vi "ExSubAsyncColDispStr.vi"(2 "error in (no error)":errorcluster, 3 "Store Data":bool, 4 "Display Title":string, 5 "Handle Cluster":T1) -> (0 "error out":errorcluster, 1 "Handle Cluster Out":T1)   [LabVIEW 2010]
panel:
  # "ExSubAsyncColDispStr:\nThis Sub-VI does the data collection, \ndisplay, and storage for Async\ncamera operations."
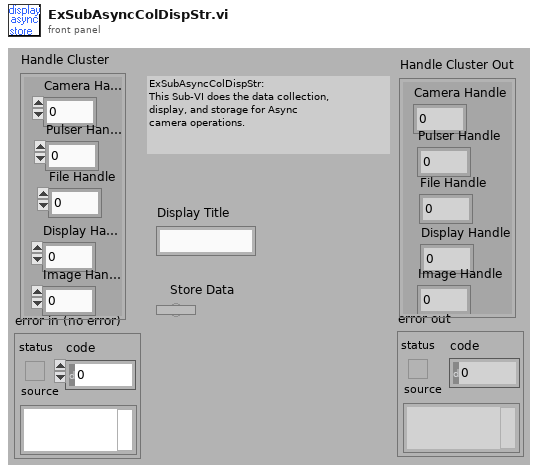
[diagram p1: front panel]
types:
  T1 = cluster{"Camera Handle":u32, "Pulser Handle":u32, "File Handle":u32, "Display Handle":u32, "Image Handle":u32}
  T2 = cluster{"Camera Handle":u32, "Pulser Handle":u32, "File Handle":u32, "Display Handle":u32, "Data Handle":u32}
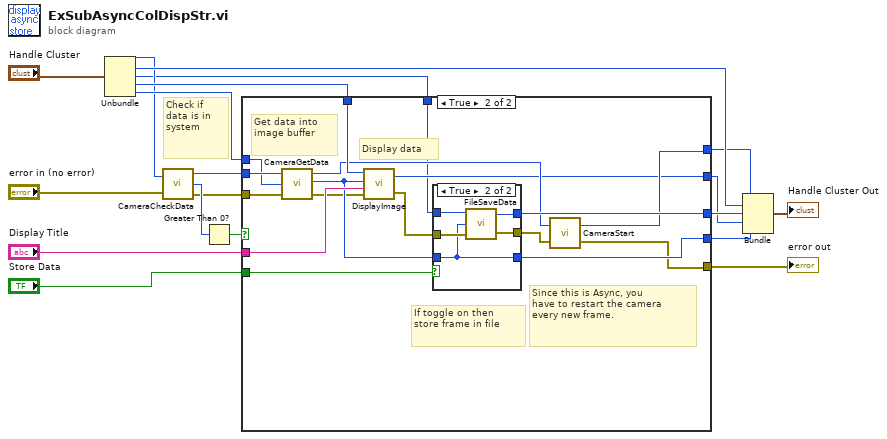
[diagram p0: block diagram]
diagram:
  # "Check if \ndata is in\nsystem"
  n1 = Unbundle("Handle Cluster") -> ("Camera Handle"=w6:u32, "Pulser Handle"=w9:u32, "File Handle"=w1:u32, "Display Handle"=w11:u32, "Image Handle"=w12:u32)
  n2 = call <userlib>:"CameraCheckData.vi"("Camera Handle"=w6, "error in"="error in (no error)") -> ("Camera Handle"=w16:u32, "Number Of Frames Available"=w15:i32, "error out"=w14:errorcluster)
  n3 = Greater Than 0?(x=w15) -> (x > 0?=w17:bool)
  n4 = case shown="True" w17 {
    tunnel: w16 -> [w24 w41]
    tunnel: w14 -> [w23 w40]
    tunnel: w12 -> [w21 w38]
    tunnel: w11 -> [w22 w37]
    tunnel: [w24 w28] -> w7
    tunnel: [w20 w39] -> w5
    tunnel: "Display Title" -> [_ w36]
    tunnel: w1 -> [w20 w25]
    tunnel: [w22 w26] -> w4
    tunnel: [w23 w29] -> w8
    tunnel: [w21 w34] -> w3
    tunnel: "Store Data" -> [_ w33]
    frame False {
    }
    frame True {
      # "If toggle on then\nstore frame in file"
      # "Since this is Async, you\nhave to restart the camera\nevery new frame."
      # "Display data"
      # "Get data into\nimage buffer"
      n5 = call <userlib>:"CameraGetData.vi"("error in"=w40, "Data Handle"=w38, "Camera Handle"=w41) -> ("error out"=w32:errorcluster, "Data Handle"=w35:u32, "Camera Handle"=w27:u32)
      n6 = call <userlib>:"DisplayImage.vi"("error in"=w32, "Title"=w36, "Image Handle"=w35, "Display Handle"=w37) -> ("error out"=w31:errorcluster, "Display Handle"=w26:u32)
      n7 = case shown="True" w33 {
        tunnel: [w44 w49] -> w39
        tunnel: w31 -> [w43 w48]
        tunnel: w25 -> [w44 w45]
        tunnel: [w43 w47] -> w30
        tunnel: w35 -> [w42 w46]
        tunnel: [w42 w46] -> w34
        frame False {
        }
        frame True {
          n8 = call <userlib>:"FileSaveData.vi"("error in"=w48, "Image Handle"=w46, "File Handle"=w45) -> ("error out"=w47:errorcluster, "File Handle"=w49:u32)
        }
      }
      n9 = call <userlib>:"CameraStart.vi"("error in"=w30, "Camera Handle"=w27) -> ("error out"=w29:errorcluster, "Camera Handle"=w28:u32)
    }
  }
  "error out" <- w8
  n10 = Bundle("Camera Handle"=w7, "Pulser Handle"=w9, "File Handle"=w5, "Display Handle"=w4, "Data Handle"=w3) -> (→"Handle Cluster Out":T2)  [unwired: 1 in]
